vi "filter_calcs.vi"(8 "Detector 3 Correlations In":T1, 9 "Detector 1 Correlations In":T1, 10 "Detector 3":i16, 11 "Detector 1":i16) -> (0 "Detector 3 Correlations Out":T1, 1 "Detector 1 Correlations Out":T1)   [LabVIEW 2015]
uses:
  Detector_Cluster.ctl
  <vilib>/rvi/Emulation/niFpgaSctlEmulationGetInTimedLoop.vi
  <vilib>/Utility/error.llb/Clear Errors.vi
  <vilib>/rvi/Emulation/niFpgaEmulationIsFPGAContextNoSignature.vi
  <vilib>/rvi/errors/niFpgaSetErrorForExecOnDevCompSimple.vi
  <vilib>/rvi/eio/common/nirviEmuReportErrorAndStop.vi
  <vilib>/rvi/DataTransferAndStorage/Container/Common/niFpgaContainerGetUniqueNameForEmu.vi
  <vilib>/rvi/FIFO/Fifo_Resource/nirvififoEmulationSetSize.vi
  <vilib>/rvi/FIFO/Fifo_Resource/nirviFifoEmulationQueueMgr.vi
  <instcachedir>/0/nirviFifoEmulationQueueMgr_E5CAEC123FF24DC58D834DCA3CDAA9B5.lvgen/nirviFifoEmulationQueueMgr_E5CAEC123FF24DC58D834DCA3CDAA9B5_002.vi
  <vilib>/rvi/FIFO/Fifo_Resource/nirvififoEmulationDetermineInputValidOut.vi
  <vilib>/rvi/FIFO/Fifo_Resource/nirvififoEmulationCreateLock.vi
  <vilib>/rvi/Emulation/niFpgaProcessEmulError.vi
  <vilib>/rvi/FIFO/Fifo_Resource/nirvififoEmulationObtainLock.vi
  <vilib>/rvi/FIFO/Fifo_Resource/nirvififoEmulationReleaseLock.vi
  <vilib>/rvi/occurrence/nirviWaitOnOccurrenceBase.vi
  <vilib>/rvi/errors/nirviReportUnexpectedCaseInternalError.vi
  <vilib>/rvi/errors/nirviReportUnexpectedCaseInternalError (U32).vi
  <vilib>/rvi/DataTransferAndStorage/Container/Common/niFpgaContainerExecOnDevCompGetState.vi
  <vilib>/rvi/interface/RandomDataEmulation/niFpgaRandomDataHandleErrors.vi
  <vilib>/rvi/DataTransferAndStorage/Container/XNode/niFpgaContainer.xnode
  <vilib>/rvi/FIFO/Fifo_Resource/nirvififoEmulationWrite.vi
  <vilib>/rvi/FIFO/Fifo_Resource/niFpgaFifoEmulationRefIn.vi
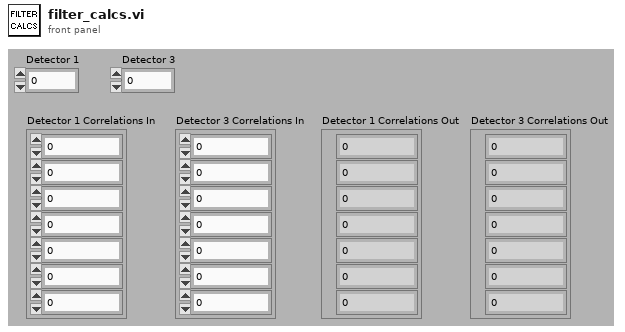
[diagram p1: front panel]
types:
  T1 = typedef "Detector_Cluster.ctl" = cluster{"1":i32, "2":i32, "3":i32, "4":i32, "5":i32, "6":i32, "7":i32}
  T2 = cluster{"Average Out":i32, "Next State":u16, "Detector 1 Correlation out":i32, "Detector 3 Correlation out":i32, "Velocity Count out":i32, "Detector counter out":i32, "Timeout count out":u32}
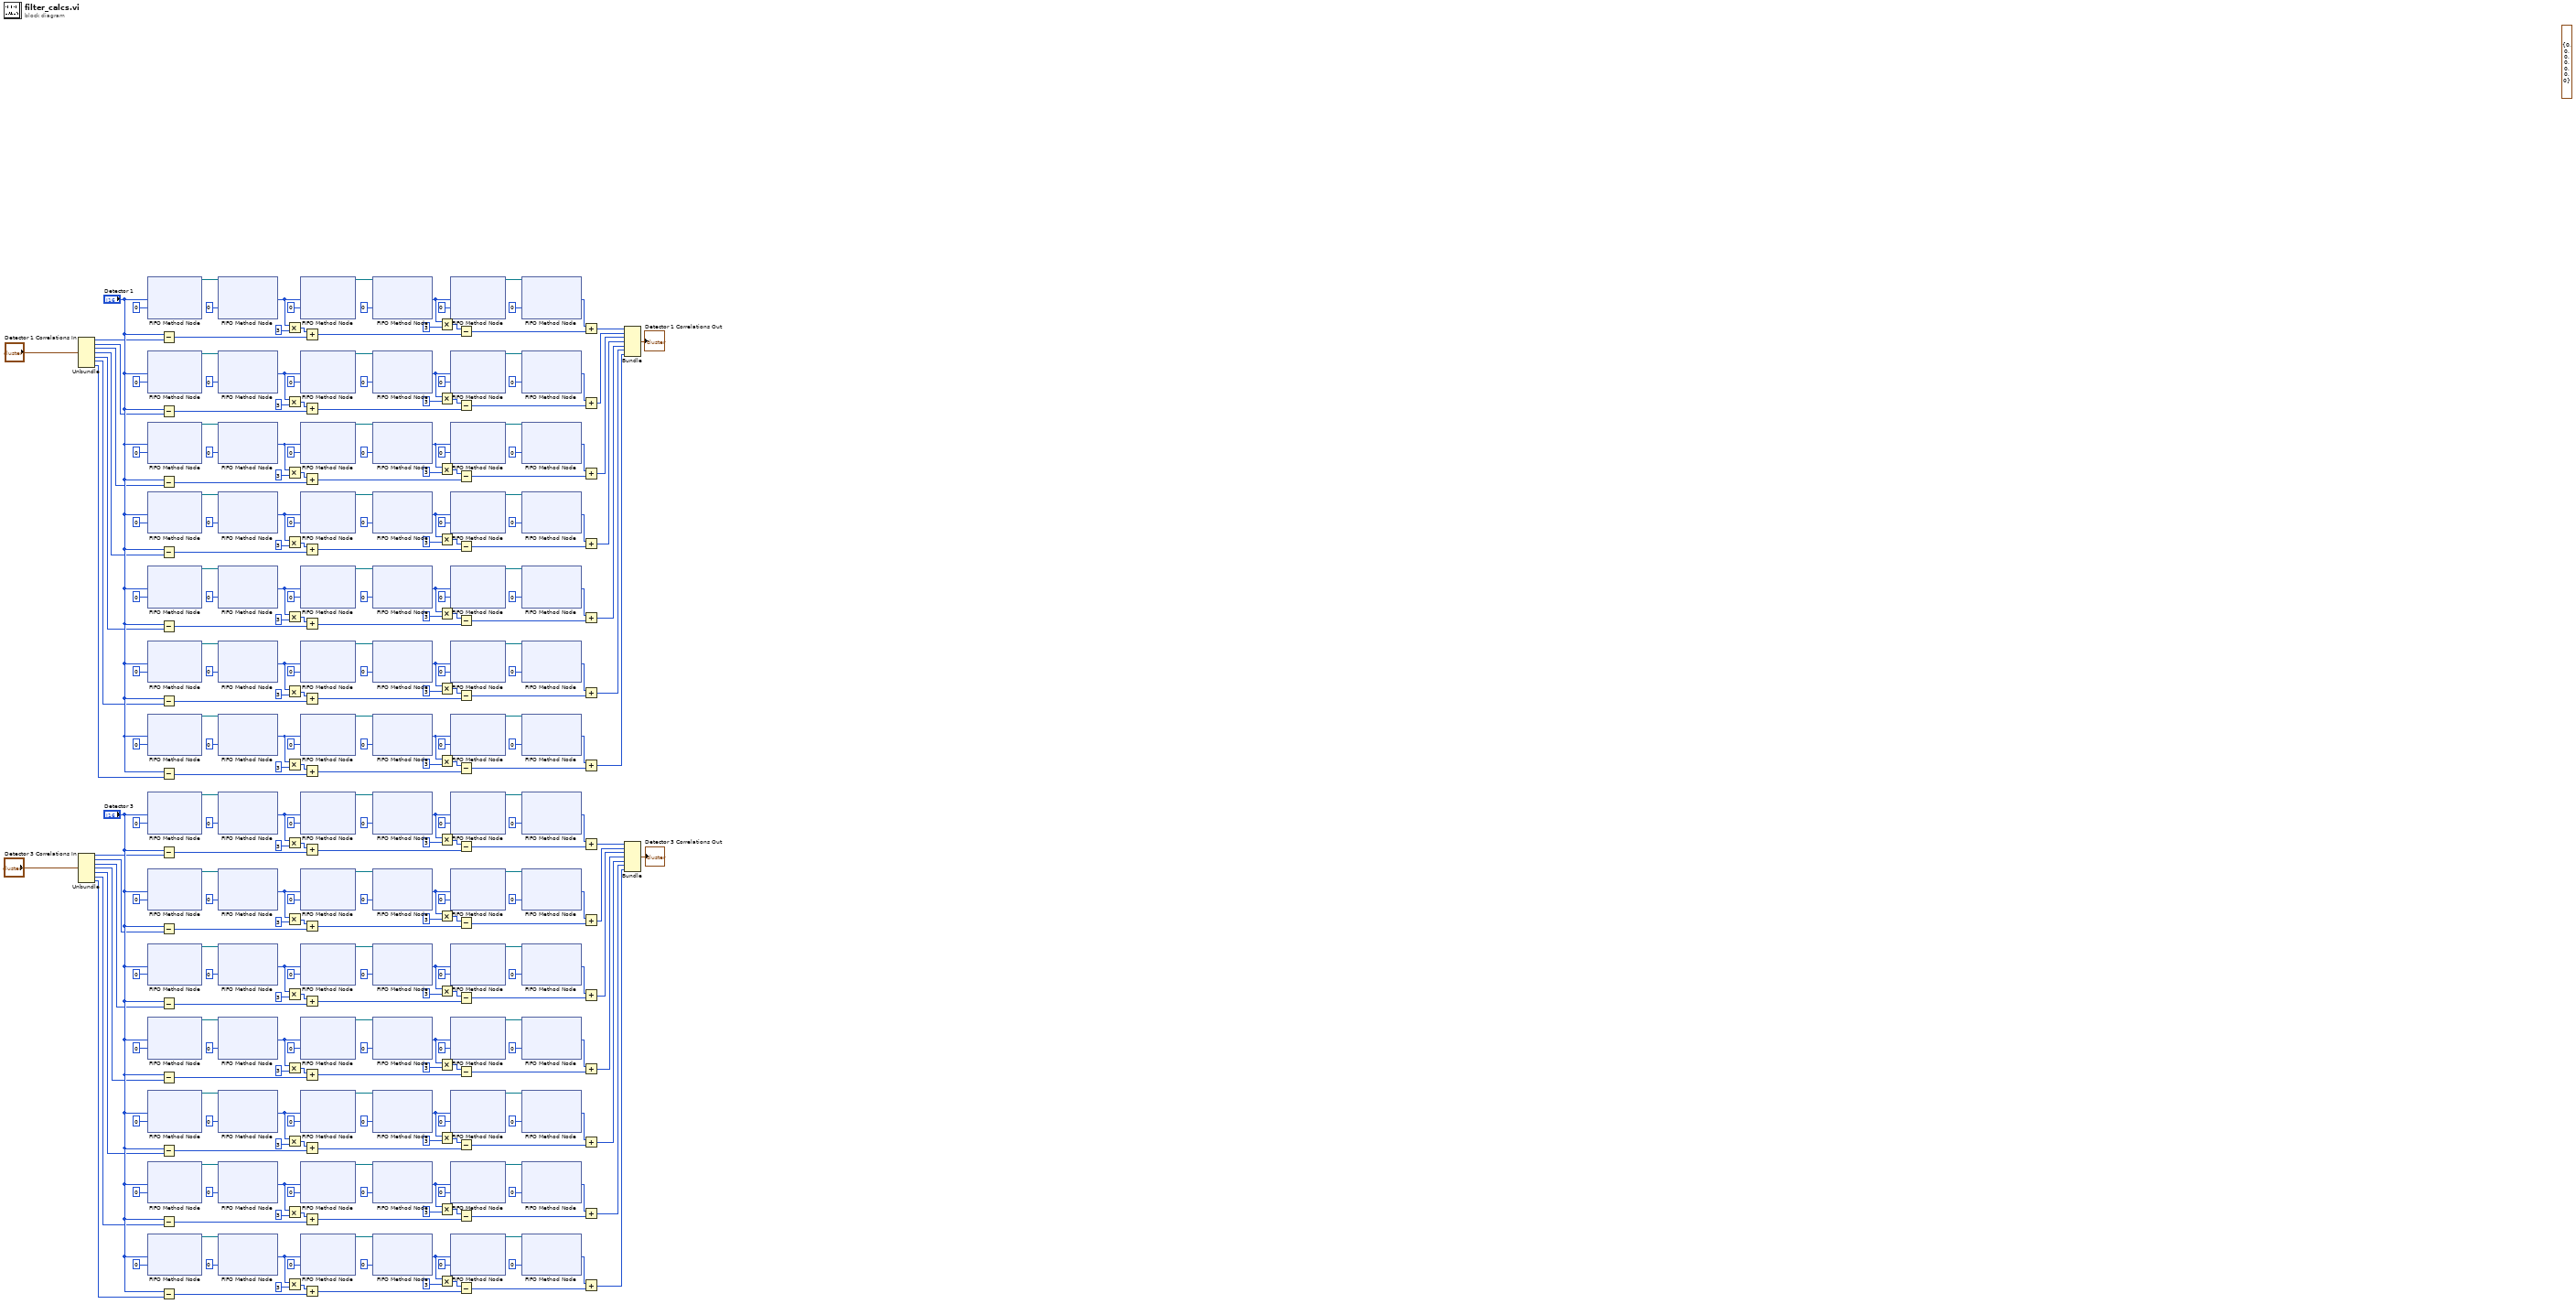
[diagram p0: block diagram]
diagram:
  (unwired) T2 {"Average Out"=0, "Next State"=0, "Detector 1 Correlation out"=0, "Detector 3 Correlation out"=0, "Velocity Count out"=0, "Detector counter out"=0, "Timeout count out"=0} ("Output Cluster")
  n1 = Unbundle("Detector 1 Correlations In") -> ("1"=w24:i32, "2"=w17:i32, "3"=w18:i32, "4"=w19:i32, "5"=w20:i32, "6"=w21:i32, "7"=w22:i32)
  n2 = Unbundle("Detector 3 Correlations In") -> ("1"=w31:i32, "2"=w25:i32, "3"=w26:i32, "4"=w27:i32, "5"=w28:i32, "6"=w29:i32, "7"=w30:i32)
  n3 = xnode ("FIFO Method Node")("Element"="Detector 1", "Timeout"=0) -> ("FIFO Out"=w250:refnum<k21>)  [unwired: 1 in, 1 out]
  n4 = xnode ("FIFO Method Node")("Element"="Detector 1", "Timeout"=0) -> ("FIFO Out"=w275:refnum<k21>)  [unwired: 1 in, 1 out]
  n5 = xnode ("FIFO Method Node")("Element"="Detector 1", "Timeout"=0) -> ("FIFO Out"=w288:refnum<k21>)  [unwired: 1 in, 1 out]
  n6 = xnode ("FIFO Method Node")("Element"="Detector 1", "Timeout"=0) -> ("FIFO Out"=w237:refnum<k21>)  [unwired: 1 in, 1 out]
  n7 = xnode ("FIFO Method Node")("Element"="Detector 1", "Timeout"=0) -> ("FIFO Out"=w212:refnum<k21>)  [unwired: 1 in, 1 out]
  n8 = xnode ("FIFO Method Node")("Element"="Detector 1", "Timeout"=0) -> ("FIFO Out"=w199:refnum<k21>)  [unwired: 1 in, 1 out]
  n9 = xnode ("FIFO Method Node")("Element"="Detector 1", "Timeout"=0) -> ("FIFO Out"=w174:refnum<k21>)  [unwired: 1 in, 1 out]
  n10 = xnode ("FIFO Method Node")("Element"="Detector 3", "Timeout"=0) -> ("FIFO Out"=w161:refnum<k21>)  [unwired: 1 in, 1 out]
  n11 = xnode ("FIFO Method Node")("Element"="Detector 3", "Timeout"=0) -> ("FIFO Out"=w136:refnum<k21>)  [unwired: 1 in, 1 out]
  n12 = xnode ("FIFO Method Node")("Element"="Detector 3", "Timeout"=0) -> ("FIFO Out"=w123:refnum<k21>)  [unwired: 1 in, 1 out]
  n13 = xnode ("FIFO Method Node")("Element"="Detector 3", "Timeout"=0) -> ("FIFO Out"=w98:refnum<k21>)  [unwired: 1 in, 1 out]
  n14 = xnode ("FIFO Method Node")("Element"="Detector 3", "Timeout"=0) -> ("FIFO Out"=w85:refnum<k21>)  [unwired: 1 in, 1 out]
  n15 = xnode ("FIFO Method Node")("Element"="Detector 3", "Timeout"=0) -> ("FIFO Out"=w60:refnum<k21>)  [unwired: 1 in, 1 out]
  n16 = xnode ("FIFO Method Node")("Element"="Detector 3", "Timeout"=0) -> ("FIFO Out"=w47:refnum<k21>)  [unwired: 1 in, 1 out]
  n17 = Subtract(x="Detector 1", y=w24) -> (x-y=w262:i32)
  n18 = Subtract(x="Detector 1", y=w17) -> (x-y=w263:i32)
  n19 = Subtract(x="Detector 1", y=w18) -> (x-y=w300:i32)
  n20 = Subtract(x="Detector 1", y=w19) -> (x-y=w225:i32)
  n21 = Subtract(x="Detector 1", y=w20) -> (x-y=w224:i32)
  n22 = Subtract(x="Detector 1", y=w21) -> (x-y=w187:i32)
  n23 = Subtract(x="Detector 1", y=w22) -> (x-y=w186:i32)
  n24 = Subtract(x="Detector 3", y=w31) -> (x-y=w149:i32)
  n25 = Subtract(x="Detector 3", y=w25) -> (x-y=w148:i32)
  n26 = Subtract(x="Detector 3", y=w26) -> (x-y=w111:i32)
  n27 = Subtract(x="Detector 3", y=w27) -> (x-y=w110:i32)
  n28 = Subtract(x="Detector 3", y=w28) -> (x-y=w73:i32)
  n29 = Subtract(x="Detector 3", y=w29) -> (x-y=w72:i32)
  n30 = Subtract(x="Detector 3", y=w30) -> (x-y=w35:i32)
  n31 = xnode ("FIFO Method Node")("Timeout"=0, "FIFO In"=w250) -> ("Element"=w257:i16)  [unwired: 2 out]
  n32 = xnode ("FIFO Method Node")("Timeout"=0, "FIFO In"=w275) -> ("Element"=w268:i16)  [unwired: 2 out]
  n33 = xnode ("FIFO Method Node")("Timeout"=0, "FIFO In"=w288) -> ("Element"=w295:i16)  [unwired: 2 out]
  n34 = xnode ("FIFO Method Node")("Timeout"=0, "FIFO In"=w237) -> ("Element"=w230:i16)  [unwired: 2 out]
  n35 = xnode ("FIFO Method Node")("Timeout"=0, "FIFO In"=w212) -> ("Element"=w219:i16)  [unwired: 2 out]
  n36 = xnode ("FIFO Method Node")("Timeout"=0, "FIFO In"=w199) -> ("Element"=w192:i16)  [unwired: 2 out]
  n37 = xnode ("FIFO Method Node")("Timeout"=0, "FIFO In"=w174) -> ("Element"=w181:i16)  [unwired: 2 out]
  n38 = xnode ("FIFO Method Node")("Timeout"=0, "FIFO In"=w161) -> ("Element"=w154:i16)  [unwired: 2 out]
  n39 = xnode ("FIFO Method Node")("Timeout"=0, "FIFO In"=w136) -> ("Element"=w143:i16)  [unwired: 2 out]
  n40 = xnode ("FIFO Method Node")("Timeout"=0, "FIFO In"=w123) -> ("Element"=w116:i16)  [unwired: 2 out]
  n41 = xnode ("FIFO Method Node")("Timeout"=0, "FIFO In"=w98) -> ("Element"=w105:i16)  [unwired: 2 out]
  n42 = xnode ("FIFO Method Node")("Timeout"=0, "FIFO In"=w85) -> ("Element"=w78:i16)  [unwired: 2 out]
  n43 = xnode ("FIFO Method Node")("Timeout"=0, "FIFO In"=w60) -> ("Element"=w67:i16)  [unwired: 2 out]
  n44 = xnode ("FIFO Method Node")("Timeout"=0, "FIFO In"=w47) -> ("Element"=w40:i16)  [unwired: 2 out]
  n45 = Multiply(x=w257, y=i16 3) -> (x*y=w256:i16)
  n46 = Multiply(x=w268, y=i16 3) -> (x*y=w269:i16)
  n47 = Multiply(x=w295, y=i16 3) -> (x*y=w294:i16)
  n48 = Multiply(x=w230, y=i16 3) -> (x*y=w231:i16)
  n49 = Multiply(x=w219, y=i16 3) -> (x*y=w218:i16)
  n50 = Multiply(x=w192, y=i16 3) -> (x*y=w193:i16)
  n51 = Multiply(x=w181, y=i16 3) -> (x*y=w180:i16)
  n52 = Multiply(x=w154, y=i16 3) -> (x*y=w155:i16)
  n53 = Multiply(x=w143, y=i16 3) -> (x*y=w142:i16)
  n54 = Multiply(x=w116, y=i16 3) -> (x*y=w117:i16)
  n55 = Multiply(x=w105, y=i16 3) -> (x*y=w104:i16)
  n56 = Multiply(x=w78, y=i16 3) -> (x*y=w79:i16)
  n57 = Multiply(x=w67, y=i16 3) -> (x*y=w66:i16)
  n58 = Multiply(x=w40, y=i16 3) -> (x*y=w41:i16)
  n59 = xnode ("FIFO Method Node")("Element"=w257, "Timeout"=0) -> ("FIFO Out"=w247:refnum<k21>)  [unwired: 1 in, 1 out]
  n60 = xnode ("FIFO Method Node")("Element"=w268, "Timeout"=0) -> ("FIFO Out"=w278:refnum<k21>)  [unwired: 1 in, 1 out]
  n61 = xnode ("FIFO Method Node")("Element"=w295, "Timeout"=0) -> ("FIFO Out"=w285:refnum<k21>)  [unwired: 1 in, 1 out]
  n62 = xnode ("FIFO Method Node")("Element"=w230, "Timeout"=0) -> ("FIFO Out"=w240:refnum<k21>)  [unwired: 1 in, 1 out]
  n63 = xnode ("FIFO Method Node")("Element"=w219, "Timeout"=0) -> ("FIFO Out"=w209:refnum<k21>)  [unwired: 1 in, 1 out]
  n64 = xnode ("FIFO Method Node")("Element"=w192, "Timeout"=0) -> ("FIFO Out"=w202:refnum<k21>)  [unwired: 1 in, 1 out]
  n65 = xnode ("FIFO Method Node")("Element"=w181, "Timeout"=0) -> ("FIFO Out"=w171:refnum<k21>)  [unwired: 1 in, 1 out]
  n66 = xnode ("FIFO Method Node")("Element"=w154, "Timeout"=0) -> ("FIFO Out"=w164:refnum<k21>)  [unwired: 1 in, 1 out]
  n67 = xnode ("FIFO Method Node")("Element"=w143, "Timeout"=0) -> ("FIFO Out"=w133:refnum<k21>)  [unwired: 1 in, 1 out]
  n68 = xnode ("FIFO Method Node")("Element"=w116, "Timeout"=0) -> ("FIFO Out"=w126:refnum<k21>)  [unwired: 1 in, 1 out]
  n69 = xnode ("FIFO Method Node")("Element"=w105, "Timeout"=0) -> ("FIFO Out"=w95:refnum<k21>)  [unwired: 1 in, 1 out]
  n70 = xnode ("FIFO Method Node")("Element"=w78, "Timeout"=0) -> ("FIFO Out"=w88:refnum<k21>)  [unwired: 1 in, 1 out]
  n71 = xnode ("FIFO Method Node")("Element"=w67, "Timeout"=0) -> ("FIFO Out"=w57:refnum<k21>)  [unwired: 1 in, 1 out]
  n72 = xnode ("FIFO Method Node")("Element"=w40, "Timeout"=0) -> ("FIFO Out"=w50:refnum<k21>)  [unwired: 1 in, 1 out]
  n73 = Add(x=w256, y=w262) -> (x+y=w248:i32)
  n74 = Add(x=w269, y=w263) -> (x+y=w277:i32)
  n75 = Add(x=w294, y=w300) -> (x+y=w286:i32)
  n76 = Add(x=w231, y=w225) -> (x+y=w239:i32)
  n77 = Add(x=w218, y=w224) -> (x+y=w210:i32)
  n78 = Add(x=w193, y=w187) -> (x+y=w201:i32)
  n79 = Add(x=w180, y=w186) -> (x+y=w172:i32)
  n80 = Add(x=w155, y=w149) -> (x+y=w163:i32)
  n81 = Add(x=w142, y=w148) -> (x+y=w134:i32)
  n82 = Add(x=w117, y=w111) -> (x+y=w125:i32)
  n83 = Add(x=w104, y=w110) -> (x+y=w96:i32)
  n84 = Add(x=w79, y=w73) -> (x+y=w87:i32)
  n85 = Add(x=w66, y=w72) -> (x+y=w58:i32)
  n86 = Add(x=w41, y=w35) -> (x+y=w49:i32)
  n87 = xnode ("FIFO Method Node")("Timeout"=0, "FIFO In"=w247) -> ("Element"=w252:i16)  [unwired: 2 out]
  n88 = xnode ("FIFO Method Node")("Timeout"=0, "FIFO In"=w278) -> ("Element"=w273:i16)  [unwired: 2 out]
  n89 = xnode ("FIFO Method Node")("Timeout"=0, "FIFO In"=w285) -> ("Element"=w290:i16)  [unwired: 2 out]
  n90 = xnode ("FIFO Method Node")("Timeout"=0, "FIFO In"=w240) -> ("Element"=w235:i16)  [unwired: 2 out]
  n91 = xnode ("FIFO Method Node")("Timeout"=0, "FIFO In"=w209) -> ("Element"=w214:i16)  [unwired: 2 out]
  n92 = xnode ("FIFO Method Node")("Timeout"=0, "FIFO In"=w202) -> ("Element"=w197:i16)  [unwired: 2 out]
  n93 = xnode ("FIFO Method Node")("Timeout"=0, "FIFO In"=w171) -> ("Element"=w176:i16)  [unwired: 2 out]
  n94 = xnode ("FIFO Method Node")("Timeout"=0, "FIFO In"=w164) -> ("Element"=w159:i16)  [unwired: 2 out]
  n95 = xnode ("FIFO Method Node")("Timeout"=0, "FIFO In"=w133) -> ("Element"=w138:i16)  [unwired: 2 out]
  n96 = xnode ("FIFO Method Node")("Timeout"=0, "FIFO In"=w126) -> ("Element"=w121:i16)  [unwired: 2 out]
  n97 = xnode ("FIFO Method Node")("Timeout"=0, "FIFO In"=w95) -> ("Element"=w100:i16)  [unwired: 2 out]
  n98 = xnode ("FIFO Method Node")("Timeout"=0, "FIFO In"=w88) -> ("Element"=w83:i16)  [unwired: 2 out]
  n99 = xnode ("FIFO Method Node")("Timeout"=0, "FIFO In"=w57) -> ("Element"=w62:i16)  [unwired: 2 out]
  n100 = xnode ("FIFO Method Node")("Timeout"=0, "FIFO In"=w50) -> ("Element"=w45:i16)  [unwired: 2 out]
  n101 = Multiply(x=w252, y=i16 3) -> (x*y=w249:i16)
  n102 = Multiply(x=w273, y=i16 3) -> (x*y=w276:i16)
  n103 = Multiply(x=w290, y=i16 3) -> (x*y=w287:i16)
  n104 = Multiply(x=w235, y=i16 3) -> (x*y=w238:i16)
  n105 = Multiply(x=w214, y=i16 3) -> (x*y=w211:i16)
  n106 = Multiply(x=w197, y=i16 3) -> (x*y=w200:i16)
  n107 = Multiply(x=w176, y=i16 3) -> (x*y=w173:i16)
  n108 = Multiply(x=w159, y=i16 3) -> (x*y=w162:i16)
  n109 = Multiply(x=w138, y=i16 3) -> (x*y=w135:i16)
  n110 = Multiply(x=w121, y=i16 3) -> (x*y=w124:i16)
  n111 = Multiply(x=w100, y=i16 3) -> (x*y=w97:i16)
  n112 = Multiply(x=w83, y=i16 3) -> (x*y=w86:i16)
  n113 = Multiply(x=w62, y=i16 3) -> (x*y=w59:i16)
  n114 = Multiply(x=w45, y=i16 3) -> (x*y=w48:i16)
  n115 = xnode ("FIFO Method Node")("Element"=w252, "Timeout"=0) -> ("FIFO Out"=w246:refnum<k21>)  [unwired: 1 in, 1 out]
  n116 = xnode ("FIFO Method Node")("Element"=w273, "Timeout"=0) -> ("FIFO Out"=w279:refnum<k21>)  [unwired: 1 in, 1 out]
  n117 = xnode ("FIFO Method Node")("Element"=w290, "Timeout"=0) -> ("FIFO Out"=w284:refnum<k21>)  [unwired: 1 in, 1 out]
  n118 = xnode ("FIFO Method Node")("Element"=w235, "Timeout"=0) -> ("FIFO Out"=w241:refnum<k21>)  [unwired: 1 in, 1 out]
  n119 = xnode ("FIFO Method Node")("Element"=w214, "Timeout"=0) -> ("FIFO Out"=w208:refnum<k21>)  [unwired: 1 in, 1 out]
  n120 = xnode ("FIFO Method Node")("Element"=w197, "Timeout"=0) -> ("FIFO Out"=w203:refnum<k21>)  [unwired: 1 in, 1 out]
  n121 = xnode ("FIFO Method Node")("Element"=w176, "Timeout"=0) -> ("FIFO Out"=w170:refnum<k21>)  [unwired: 1 in, 1 out]
  n122 = xnode ("FIFO Method Node")("Element"=w159, "Timeout"=0) -> ("FIFO Out"=w165:refnum<k21>)  [unwired: 1 in, 1 out]
  n123 = xnode ("FIFO Method Node")("Element"=w138, "Timeout"=0) -> ("FIFO Out"=w132:refnum<k21>)  [unwired: 1 in, 1 out]
  n124 = xnode ("FIFO Method Node")("Element"=w121, "Timeout"=0) -> ("FIFO Out"=w127:refnum<k21>)  [unwired: 1 in, 1 out]
  n125 = xnode ("FIFO Method Node")("Element"=w100, "Timeout"=0) -> ("FIFO Out"=w94:refnum<k21>)  [unwired: 1 in, 1 out]
  n126 = xnode ("FIFO Method Node")("Element"=w83, "Timeout"=0) -> ("FIFO Out"=w89:refnum<k21>)  [unwired: 1 in, 1 out]
  n127 = xnode ("FIFO Method Node")("Element"=w62, "Timeout"=0) -> ("FIFO Out"=w56:refnum<k21>)  [unwired: 1 in, 1 out]
  n128 = xnode ("FIFO Method Node")("Element"=w45, "Timeout"=0) -> ("FIFO Out"=w51:refnum<k21>)  [unwired: 1 in, 1 out]
  n129 = Subtract(x=w249, y=w248) -> (x-y=w244:i32)
  n130 = Subtract(x=w276, y=w277) -> (x-y=w281:i32)
  n131 = Subtract(x=w287, y=w286) -> (x-y=w282:i32)
  n132 = Subtract(x=w238, y=w239) -> (x-y=w243:i32)
  n133 = Subtract(x=w211, y=w210) -> (x-y=w206:i32)
  n134 = Subtract(x=w200, y=w201) -> (x-y=w205:i32)
  n135 = Subtract(x=w173, y=w172) -> (x-y=w168:i32)
  n136 = Subtract(x=w162, y=w163) -> (x-y=w167:i32)
  n137 = Subtract(x=w135, y=w134) -> (x-y=w130:i32)
  n138 = Subtract(x=w124, y=w125) -> (x-y=w129:i32)
  n139 = Subtract(x=w97, y=w96) -> (x-y=w92:i32)
  n140 = Subtract(x=w86, y=w87) -> (x-y=w91:i32)
  n141 = Subtract(x=w59, y=w58) -> (x-y=w54:i32)
  n142 = Subtract(x=w48, y=w49) -> (x-y=w53:i32)
  n143 = xnode ("FIFO Method Node")("Timeout"=0, "FIFO In"=w246) -> ("Element"=w245:i16)  [unwired: 2 out]
  n144 = xnode ("FIFO Method Node")("Timeout"=0, "FIFO In"=w279) -> ("Element"=w280:i16)  [unwired: 2 out]
  n145 = xnode ("FIFO Method Node")("Timeout"=0, "FIFO In"=w284) -> ("Element"=w283:i16)  [unwired: 2 out]
  n146 = xnode ("FIFO Method Node")("Timeout"=0, "FIFO In"=w241) -> ("Element"=w242:i16)  [unwired: 2 out]
  n147 = xnode ("FIFO Method Node")("Timeout"=0, "FIFO In"=w208) -> ("Element"=w207:i16)  [unwired: 2 out]
  n148 = xnode ("FIFO Method Node")("Timeout"=0, "FIFO In"=w203) -> ("Element"=w204:i16)  [unwired: 2 out]
  n149 = xnode ("FIFO Method Node")("Timeout"=0, "FIFO In"=w170) -> ("Element"=w169:i16)  [unwired: 2 out]
  n150 = xnode ("FIFO Method Node")("Timeout"=0, "FIFO In"=w165) -> ("Element"=w166:i16)  [unwired: 2 out]
  n151 = xnode ("FIFO Method Node")("Timeout"=0, "FIFO In"=w132) -> ("Element"=w131:i16)  [unwired: 2 out]
  n152 = xnode ("FIFO Method Node")("Timeout"=0, "FIFO In"=w127) -> ("Element"=w128:i16)  [unwired: 2 out]
  n153 = xnode ("FIFO Method Node")("Timeout"=0, "FIFO In"=w94) -> ("Element"=w93:i16)  [unwired: 2 out]
  n154 = xnode ("FIFO Method Node")("Timeout"=0, "FIFO In"=w89) -> ("Element"=w90:i16)  [unwired: 2 out]
  n155 = xnode ("FIFO Method Node")("Timeout"=0, "FIFO In"=w56) -> ("Element"=w55:i16)  [unwired: 2 out]
  n156 = xnode ("FIFO Method Node")("Timeout"=0, "FIFO In"=w51) -> ("Element"=w52:i16)  [unwired: 2 out]
  n157 = Add(x=w245, y=w244) -> (x+y=w16:i32)
  n158 = Add(x=w280, y=w281) -> (x+y=w10:i32)
  n159 = Add(x=w283, y=w282) -> (x+y=w11:i32)
  n160 = Add(x=w242, y=w243) -> (x+y=w12:i32)
  n161 = Add(x=w207, y=w206) -> (x+y=w13:i32)
  n162 = Add(x=w204, y=w205) -> (x+y=w14:i32)
  n163 = Add(x=w169, y=w168) -> (x+y=w15:i32)
  n164 = Add(x=w166, y=w167) -> (x+y=w8:i32)
  n165 = Add(x=w131, y=w130) -> (x+y=w2:i32)
  n166 = Add(x=w128, y=w129) -> (x+y=w3:i32)
  n167 = Add(x=w93, y=w92) -> (x+y=w4:i32)
  n168 = Add(x=w90, y=w91) -> (x+y=w5:i32)
  n169 = Add(x=w55, y=w54) -> (x+y=w6:i32)
  n170 = Add(x=w52, y=w53) -> (x+y=w7:i32)
  n171 = Bundle(w16, w10, w11, w12, w13, w14, w15) -> (→"Detector 1 Correlations Out":cluster{i32, i32, i32, i32, i32, i32, i32})  [unwired: 1 in]
  n172 = Bundle(w8, w2, w3, w4, w5, w6, w7) -> (→"Detector 3 Correlations Out":cluster{i32, i32, i32, i32, i32, i32, i32})  [unwired: 1 in]
